vi "NHQ203M Open.vi"(3 "VISA resource name":refnum<visa-resource-name>="COM3") -> (0 "Error out":errorcluster, 1 "VISA out":refnum<visa-resource-name>)   [LabVIEW 2018]
uses:
  <vilib>/Utility/error.llb/DialogType.ctl
  <vilib>/Instr/_visa.llb/VISA Configure Serial Port (Instr).vi
panel:
  out "substring before match":string
  out "read buffer":string
  out "return count":u32
  out "message 2":string=" INSTRUCTIONS:\r\rNormal Use:  When using subVIs that incorporate the error in/error out (or error I/O) structure, place this handler where you want to inform the user of an error, typically at the end of the I/O data path, as the last action of the program.  If the error in error? is ERROR, the handler creates a message describing the error and its source.  If the type of dialog = 1 (default), the message is displayed to the user, who can only acknowedge it.  If the type = 2, the user can acknowledge the message or abort execution; aborting a program with active I/O is not recommended.  If the type = 0, no message is displayed; this is used to process the error programmatically, and the error out cluster elements are wired to individual terminals for that reason.  \r\rOther Use:\n\r\nlocal testing.  To test the error code of a subVI or function that does not have the error I/O structure, you can wire its error code and a source string to the local error code and error source inputs.  If error in error? indicates no error and error code is not equal to 0, the local code and source are substituted for the error in values, and error? is set TRUE (ERROR)."
  out "message":string=" INSTRUCTIONS:\r\rNormal Use:  When using subVIs that incorporate the error in/error out (or error I/O) structure, place this handler where you want to inform the user of an error, typically at the end of the I/O data path, as the last action of the program.  If the error in error? is ERROR, the handler creates a message describing the error and its source.  If the type of dialog = 1 (default), the message is displayed to the user, who can only acknowedge it.  If the type = 2, the user can acknowledge the message or abort execution; aborting a program with active I/O is not recommended.  If the type = 0, no message is displayed; this is used to process the error programmatically, and the error out cluster elements are wired to individual terminals for that reason.  \r\rOther Use:\n\r\nlocal testing.  To test the error code of a subVI or function that does not have the error I/O structure, you can wire its error code and a source string to the local error code and error source inputs.  If error in error? indicates no error and error code is not equal to 0, the local code and source are substituted for the error in values, and error? is set TRUE (ERROR)."
  out "Initial Config Read Buffer":string
  in  "Initial Configuration":string="*RST;FORM:ELEM READ;:DISP:ENAB 0;:CURR:RANG:AUTO 1;*IDN?"
  in  "XON Character":u8=17 format="%.0x"
  in  "XOFF Character":u8=19 format="%.0x"
  in  "Flow Control":u16(ring)=1 items=["None"=0, "XON/XOFF"=1, "RTS/CTS"=2, "DTR/DSR"=4]
  in  "Termination Char\n(0xA = '\\n' = LF)":u8=10 format="%.0x"
  in  "End read on termination character?":bool=TRUE
  in  "Timeout (ms)":u32=1000
  in  "Stop Bits":u16(ring)=10 items=["1.0"=10, "1.5"=15, "2.0"=20]
  in  "Parity":u16(ring) items=["None", "Odd", "Even", "Mark", "Space"]
  in  "Data Bits":u16=8 min=5 max=8 step=1
  in  "Baud Rate":u32=9600
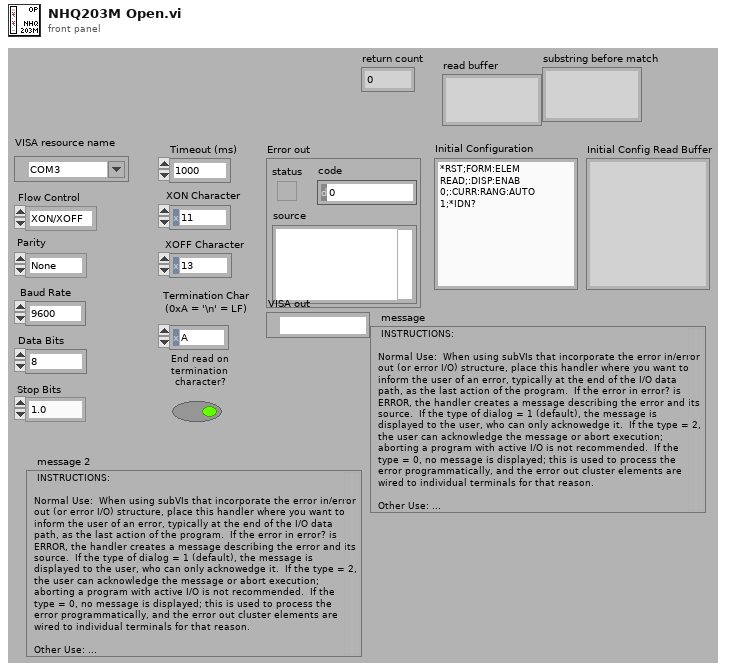
[diagram p1: front panel]
types:
  T1 = typedef "DialogType.ctl" = u16
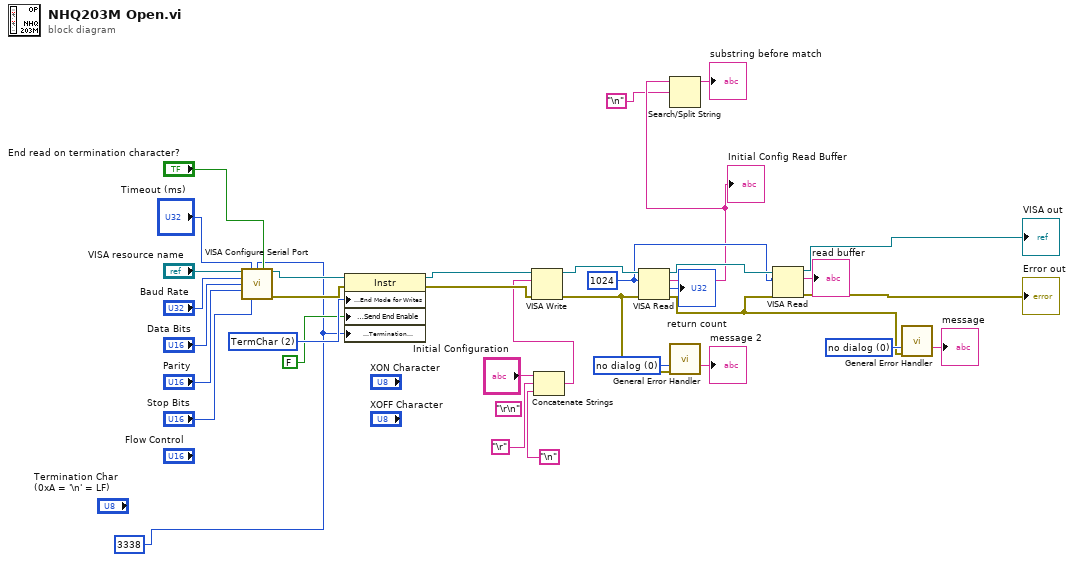
[diagram p0: block diagram]
diagram:
  w10 = 3338
  w16 = T1 0 items=["no dialog", "OK message", "continue or stop message", "OK message + warnings", "continue/stop + warnings"] ("type of dialog (OK msg:1)")
  w20 = T1 0 items=["no dialog", "OK message", "continue or stop message", "OK message + warnings", "continue/stop + warnings"] ("type of dialog (OK msg:1)")
  (unwired) "\r\n"
  w7 = u32 1024 ("byte count")
  w26 = u16 2 items=["None", "LastBit", "TermChar", "Break"] ("Serial Settings:Serial End Mode for Writes")
  n1 = call-poly "VISA Configure Serial Port"("VISA resource name"="VISA resource name", "timeout (10sec)"="Timeout (ms)", "termination char\n(0xA = '\\n' = LF)"=w10, "Enable Termination\nChar (T)"="End read on termination character?", "baud rate (9600)"="Baud Rate", "data bits (8)"="Data Bits", "parity (0:none)"="Parity", "stop bits (10: 1 bit)"="Stop Bits") -> ("VISA resource name out"=w28:refnum<visa-resource-name>, "error out"=w27:errorcluster)  [unwired: 2 in, 4 out]
  n2 = property on="Property Node" class="Instr"(reference=w28, error in=w27, "Serial Settings:End Mode for Writes"=w26, "Message Based Settings:Send End Enable"=FALSE, "Message Based Settings:Termination Character"=w10) -> (reference out=w19:refnum<visa-resource-name>, error out=w24:errorcluster)
  n3 = Concatenate Strings("Initial Configuration", "\r", "\n") -> (w22:string)
  n4 = VISA Write(VISA resource name=w19, write buffer=w22, error in (no error)=w24) -> (VISA resource name out=w29:refnum<visa-resource-name>, error out=w17:errorcluster)  [unwired: 1 out]
  n5 = VISA Read(VISA resource name=w29, byte count=w7, error in (no error)=w17) -> (VISA resource name out=w9:refnum<visa-resource-name>, read buffer=w3:string, return count=→"return count":u32, error out=w4:errorcluster)
  "Initial Config Read Buffer" <- w3
  n6 = Search/Split String(string=w3, search string/char (-)="\n") -> (substring before match=→"substring before match":string)  [unwired: 1 in, 2 out]
  n7 = call <vilib>:"General Error Handler.vi"("type of dialog (OK msg:1)"=w16, "error in (no error)"=w17) -> ("message"=→"message 2":string)  [unwired: 9 in, 4 out]
  n8 = VISA Read(VISA resource name=w9, byte count=w7, error in (no error)=w4) -> (VISA resource name out=→"VISA out":refnum<visa-resource-name>, read buffer=→"read buffer":string, error out=→"Error out":errorcluster)  [unwired: 1 out]
  n9 = call <vilib>:"General Error Handler.vi"("type of dialog (OK msg:1)"=w20, "error in (no error)"=w4) -> ("message"=→"message":string)  [unwired: 9 in, 4 out]
